vi "Lookup Channel.vi"(8 "error in (no error)":errorcluster, 10 "Channel Name":string, 11 "Group in":refnum<class "Group DBL.lvclass">) -> (0 "error out":errorcluster, 2 "Channel":refnum<class "Channel DBL.lvclass">, 3 "Group out":refnum<class "Group DBL.lvclass">)   [LabVIEW 2020, in "Vecto.lvlib" / "Group DBL.lvclass"]
uses:
  Group DBL.lvclass
  C:/dev/lv20CE/relink/lv-vecto/Vecto/Group/Group.lvclass
  Channel DBL/Channel DBL.lvclass
  Channel DBL/Channel DBL.lvclass/Channel DBL.ctl
  Group/Group.lvclass/Group.ctl
  Group Config/Group Config.lvclass/Group Config.ctl
  Group Config/Group Config.lvclass
  Group/Group.lvclass
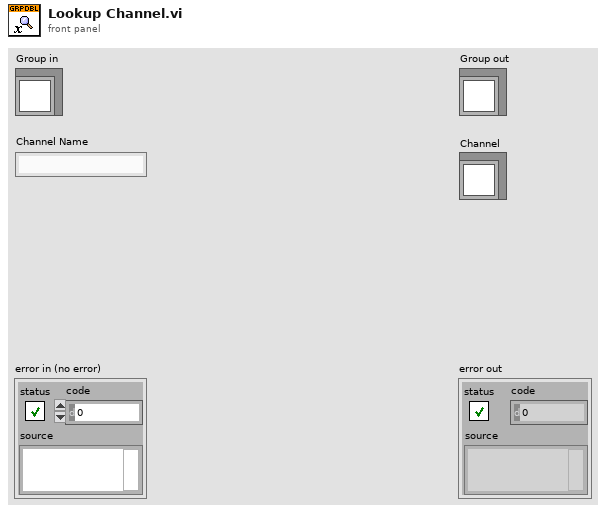
[diagram p1: front panel]
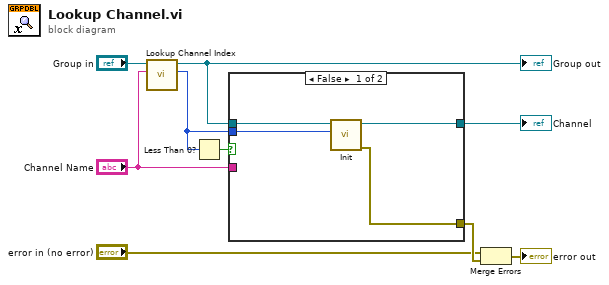
[diagram p0: block diagram]
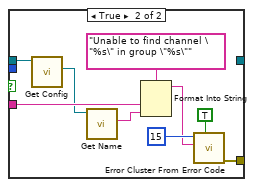
[diagram p2: hidden frame]
diagram:
  n1 = call "Lookup Channel Index.vi"("Channel Name"="Channel Name", "GroupAbstract in"="Group in") -> ("Index"=w2:i32, "GroupAbstract out"=w4:refnum<class "Group DBL.lvclass">)  [unwired: 7 in, 1 out]
  "Group out" <- w4
  n2 = Less Than 0?(x=w2) -> (x < 0?=w1:bool)
  n3 = case shown="False" w1 {
    tunnel: "Channel Name" -> [_ w20]
    tunnel: [w13 w17] -> w9
    tunnel: [w12 _] -> w6
    tunnel: w4 -> [w11 w15]
    tunnel: w2 -> [w10 _]
    frame False {
      n4 = call "Init.vi"("Channel Index"=w10, "Group"=w11) -> ("error out"=w13:errorcluster, "Channel out"=w12:refnum<class "Channel DBL.lvclass">)  [unwired: 8 in]
    }
    frame True {
      n5 = call "Get Config.vi"("GroupAbstract in"=w15) -> ("Config"=w14:refnum<class "Group Config.lvclass">)  [unwired: 8 in, 2 out]
      n6 = call "Get Name.vi"("Group Config in"=w14) -> ("Name"=w16:string)  [unwired: 8 in, 2 out]
      n7 = Format Into String(format string="Unable to find channel \"%s\" in group \"%s\"", w20, w16) -> (resulting string=w19:string)  [unwired: 2 in, 1 out]
      n8 = call <vilib>:"Error Cluster From Error Code.vi"("show call chain? (False)"=TRUE, "error message (\"\")"=w19, "error code (0)"=15) -> ("error out"=w17:errorcluster)  [unwired: 6 in]
    }
  }
  "Channel" <- w6
  n9 = Merge Errors("error in (no error)", w9) -> (→"error out":errorcluster)
